vi "KVP Parser (Standard).vi"(4 "Values":variant[](array[variant]), 6 "Keys":string[](array[string]), 8 "Strict type matching? (F)":bool, 9 "Default Value Name (empty: label)":string, 10 "Default Value":variant, 11 "Parent Name":string) -> (0 "all found?":bool, 1 "any found?":bool, 2 "Value":variant, 3 "name out":string)   [LabVIEW 2013, in "OpenVariant.lvlib"]
doc: "***********************\nDEPRECATED METHOD KEPT FOR BACKWARD COMPATIBILITY.\nUse the \"KVP Parser (Standard).vi\" method instead for future development.\n***********************\n\nThis VI takes a default value as the input and replaces it recursively (cluster, array) with values found in key value pair arrays."
uses:
  OpenVariant.lvlib
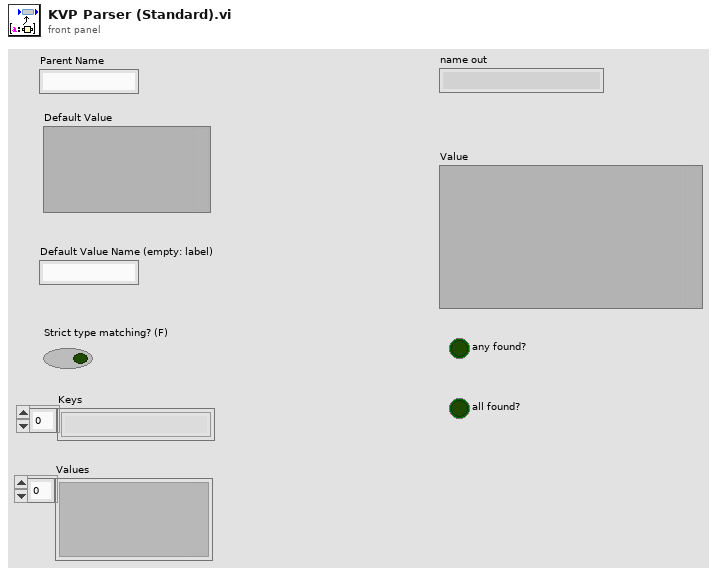
[diagram p1: front panel]
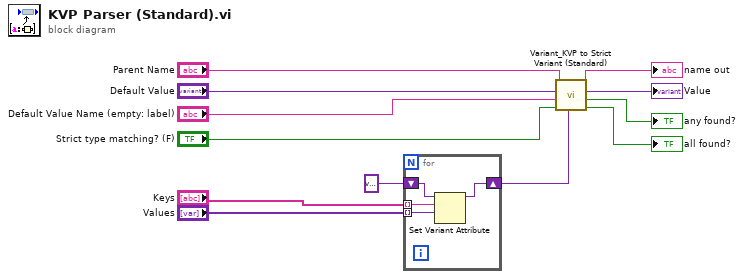
[diagram p0: block diagram]
diagram:
  n1 = for {
    tunnel: "Keys" -> [w15] mode=indexing
    tunnel: "Values" -> [w14] mode=indexing
    shift-right: [w13] -> w6
    shift-left: variant ("variant") -> [w16]
    n2 = Set Variant Attribute(Variant=w16, name=w15, value=w14) -> (Variant out=w13:variant)  [unwired: 1 in, 2 out]
  }
  n3 = call "Variant_KVP to Strict Variant (Standard).vi"("KVP"=w6, "Strict type matching? (F)"="Strict type matching? (F)", "Default Value Name (empty: label)"="Default Value Name (empty: label)", "Default Value"="Default Value", "Parent Name"="Parent Name") -> ("all found?"=→"all found?":bool, "any found?"=→"any found?":bool, "Value"=→"Value":variant, "name out"=→"name out":string)  [unwired: 3 in]
